vi "Bring Excel 2010 Window to Front_2010.vi"(3 "error in":errorcluster, 5 "Excel._Application":refnum<k7>) -> (0 "error out":errorcluster, 2 "Excel._Application":refnum<k7>)   [LabVIEW 2016, in "excel.lvlib"]
doc: "This VI uses ActiveX Automation to extract a value from the specified Worksheet and Cell range for a given excel file. If file path is empty, an windows open dialog window will appear. If the users cancels the open file, then an warning message will be sent to error handling. This VI is made specific for grabbing Dispense or Head Table excel data for the FRD. Current table formats are for 3456, 1536, and 384."
uses:
  excel.lvlib
  user32.dll
panel:
  # "Run the VI to open an instance of Excel and bring it to the front.  See the block diagram for more information on how this is accomplished."
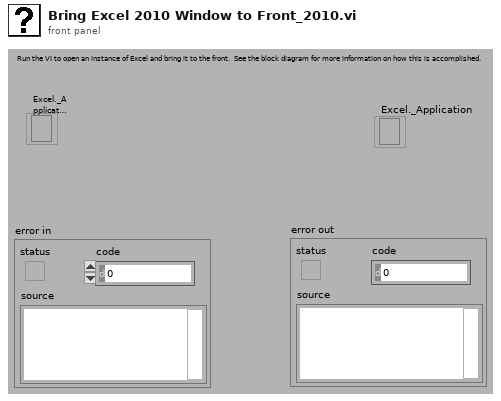
[diagram p1: front panel]
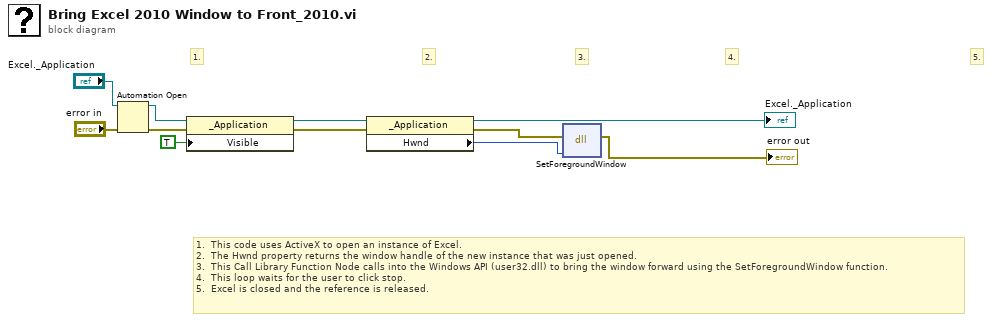
[diagram p0: block diagram]
diagram:
  # "5."
  # "1.  This code uses ActiveX to open an instance of Excel.\n2.  The Hwnd property returns the window handle of the new instance that was just opened.\n3.  This Call Library Function Node calls into the Windows API (user32.dll) to bring the window forward using the SetForegroundWindow function.\n4.  This loop waits for the user to click stop.\n5.  Excel is closed and the reference is released."
  # "3."
  # "4."
  # "2."
  # "1."
  n1 = Automation Open(error in (no error)="error in", Automation Refnum="Excel._Application") -> (Automation Refnum=w3:refnum<k7>, error out=w4:errorcluster)  [unwired: 2 in]
  n2 = property class="_Application"(reference=w3, error in=w4, "Visible"=TRUE) -> (reference out=w6:refnum<k7>, error out=w5:errorcluster)
  n3 = property class="_Application"(reference=w6, error in=w5) -> (reference out=→"Excel._Application":refnum<k7>, error out=w8:errorcluster, "Hwnd"=w10:i32)
  n4 = dll-call lib="user32.dll" fn="SetForegroundWindow"(error in=w8, "Handle"=w10) -> (error out=→"error out":errorcluster)  [unwired: 3 in, 2 out]
